vi "Inside MICAS-X Global.vi"() -> ()   [LabVIEW 2024]
panel:
  out "Inside MICAS-X?":bool
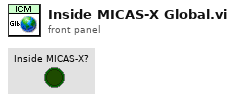
[diagram p1: front panel]
diagram:
